vi "SetGUID.vi"(0 "Interface In":refnum<class>, 1 "GUID":string, 5 "error in (no error)":errorcluster) -> (14 "Interface Out":refnum<class>, 19 "error out":errorcluster)   [LabVIEW 2016, in "GUID Trait With Attributes.lvclass"]
uses:
  GUID Trait With Attributes.lvclass
  GUID Trait With Attributes.lvclass/GUID Trait With Attributes.ctl
panel:
  # "Place Indicators here, and remember\nto connect them to the connector pane"
  # "Place Controls here, and remember\nto connect them to the connector pane"
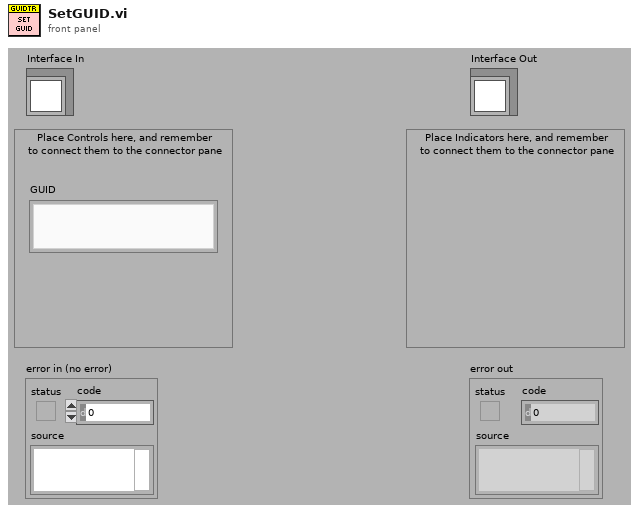
[diagram p1: front panel]
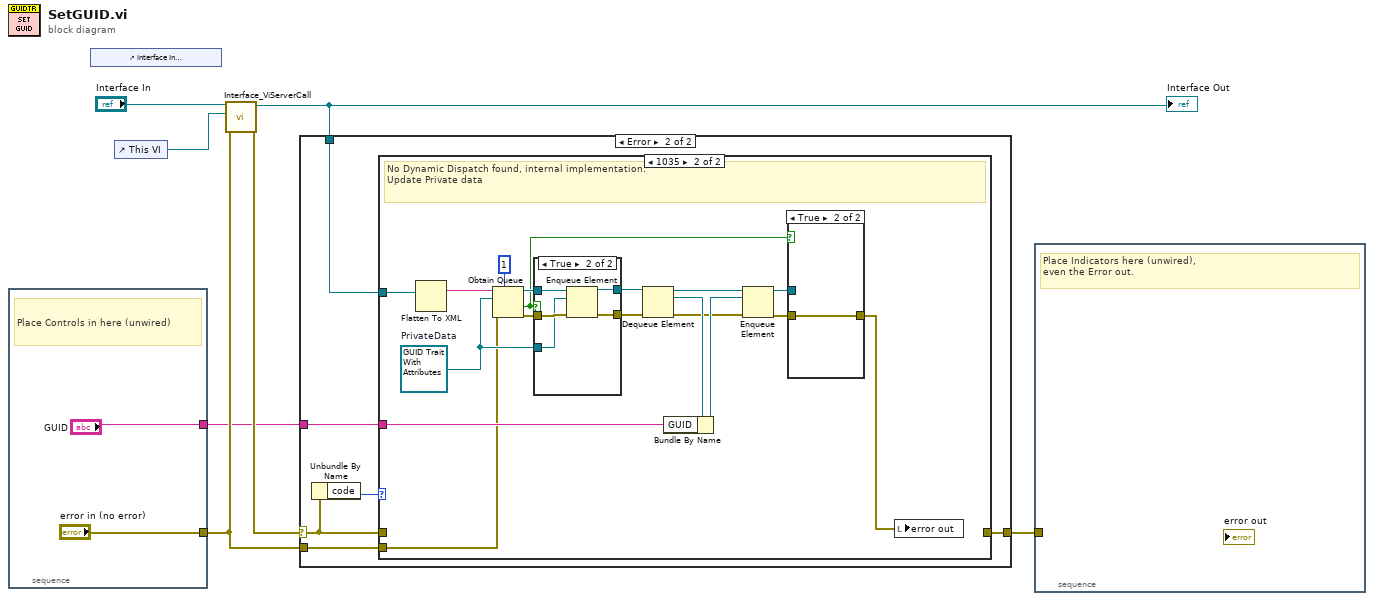
[diagram p0: block diagram]
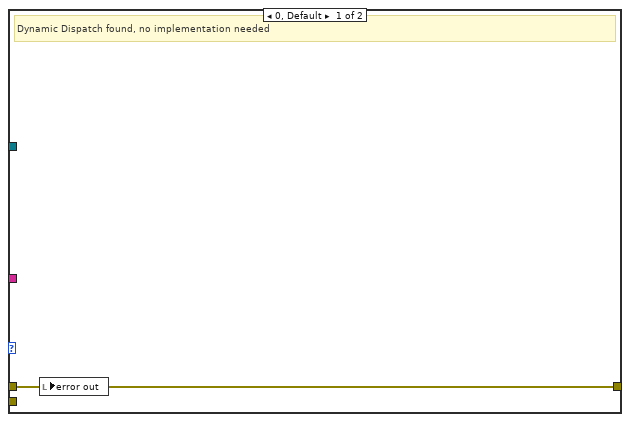
[diagram p3: hidden frame]
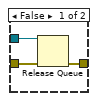
[diagram p4: hidden frame]
diagram:
  n1 = stacked-sequence {
    tunnel: ["error in (no error)"] -> w4
    tunnel: ["GUID"] -> w1
    frame #0 {
      # "Place Controls in here (unwired)"
    }
  }
  n2 = control-ref of="Interface In\nThis reference is needed to make sure this VI's front\npanel isn't removed when building an executable."() -> ()  [unwired: 1 out]
  n3 = control-ref of="This VI"() -> (w6:refnum<vi>)
  n4 = call <vilib>:"Interface_ViServerCall.vi"("error in (no error)"=w4, "Caller VI ref (This is the interface VI's reference)"=w6, "Interface In"="Interface In") -> ("error out"=w5:errorcluster, "Interface Out"=w2:refnum<class>)  [unwired: 7 in]
  "Interface Out" <- w2
  n5 = case shown="Error" w5 {
    selector: w5 -> [w10 w16]
    tunnel: [w10 w14] -> w3
    tunnel: w4 -> [_ w13]
    tunnel: w2 -> [_ w12]
    tunnel: w1 -> [_ w11]
    frame No Error {
    }
    frame Error {
      n6 = Unbundle By Name(w16) -> ("code"=w15:i32)
      n7 = case shown="1035" w15 {
        tunnel: w16 -> [w17 _]
        tunnel: [w17 _] -> w14
        tunnel: w13 -> [_ w18]
        tunnel: w12 -> [_ w35]
        tunnel: w11 -> [_ w26]
        frame 0, Default {
          # "Dynamic Dispatch found, no implementation needed"
          n8 = local write "error out"(w17) -> ()
        }
        frame 1035 {
          w31 = refnum<class "GUID Trait With Attributes.lvclass"> refnum  # PrivateData
          # "No Dynamic Dispatch found, internal implementation.\nUpdate Private data"
          n9 = Flatten To XML(anything=w35) -> (xml string=w34:string)
          n10 = Obtain Queue(max queue size (-1, unlimited)=1, name (unnamed)=w34, element data type=w31, error in (no error)=w18) -> (queue out=w33:refnum<queue>, created new?=w22:bool, error out=w32:errorcluster)  [unwired: 1 in]
          n11 = case shown="True" w22 {
            tunnel: w33 -> [w40 w46]
            tunnel: w32 -> [w41 w45]
            tunnel: w31 -> [_ w44]
            tunnel: [w40 w43] -> w29
            tunnel: [w41 w42] -> w28
            frame False {
            }
            frame True {
              n12 = Enqueue Element(queue=w46, element=w44, error in (no error)=w45) -> (queue out=w43:refnum<queue>, error out=w42:errorcluster)  [unwired: 1 in, 1 out]
            }
          }
          n13 = Dequeue Element(queue=w29, error in (no error)=w28) -> (queue out=w24:refnum<queue>, element=w27:refnum<class "GUID Trait With Attributes.lvclass">, error out=w23:errorcluster)  [unwired: 1 in, 1 out]
          n14 = Bundle By Name(cluster=w27, "GUID"=w26) -> (w25:refnum<class "GUID Trait With Attributes.lvclass">)
          n15 = Enqueue Element(queue=w24, element=w25, error in (no error)=w23) -> (queue out=w21:refnum<queue>, error out=w20:errorcluster)  [unwired: 1 in, 1 out]
          n16 = case shown="True" w22 {
            tunnel: w21 -> [w38 _]
            tunnel: w20 -> [w37 w39]
            tunnel: [w36 w39] -> w19
            frame False {
              n17 = Release Queue(queue=w38, error in (no error)=w37) -> (error out=w36:errorcluster)  [unwired: 1 in, 2 out]
            }
            frame True {
            }
          }
          n18 = local write "error out"(w19) -> ()
        }
      }
    }
  }
  n19 = stacked-sequence {
    tunnel: w3 -> [_]
    frame #0 {
      # "Place Indicators here (unwired),\neven the Error out."
    }
  }
